vi "CheckAdvancingChangeField.vi"() -> (0 "Advancing":bool)   [LabVIEW 2024]
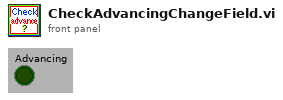
[diagram p1: front panel]
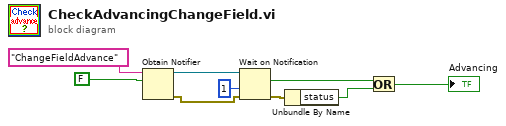
[diagram p0: block diagram]
diagram:
  n1 = Obtain Notifier(name (unnamed)="ChangeFieldAdvance", notification data type=FALSE) -> (notifier out=w8:refnum<notifier>, error out=w5:errorcluster)  [unwired: 2 in, 1 out]
  n2 = Wait on Notification(notifier=w8, timeout in ms (-1)=1, error in (no error)=w5) -> (notification=w4:bool, error out=w3:errorcluster)  [unwired: 1 in, 2 out]
  n3 = Unbundle By Name(w3) -> ("status"=w2:bool)
  n4 = Or(x=w4, y=w2) -> (x .or. y?=→"Advancing":bool)
